vi "ProdaNG.Tree.TestSteps.Add.vi"(5 "Mode":T4, 6 "FileContent":T1, 7 "TestStepsTree":refnum<vi>, 8 "error in (no error)":errorcluster, 9 "units":T5[](array[typedef]), 10 "processStepId":i32, 11 "dbHandleIn":i32) -> (0 "error out":errorcluster, 1 "#changes":i32, 3 "dbHandle":i32)   [LabVIEW 2016]
doc: "This function returns a product structure for a product, which is identified by a part and a serial number.\nImportant information: The field 'individual' was taken over from the field 'allgemein' of the legacy data directly. Because of this most products have the value 0 further on and only a few the value 1. \nParameter:\nhandle is an Integer, which is returned by the function Login() at the creation of a new connection.\nwabcoPartId is the Id of the part.\nserialNumber is the serial number of the product for the part above.\nproduct is a pointer on a product structure, which is filled if the returncode is 0. The structure must be defined in the calling program.\n\nReturncodes:\n0 No error\n< 0 ORACLE Error code\n6 (ERROR_INVALID_HANDLE) in case of an invalid handle\n1403 Record does not exist"
uses:
  Controls/ProdaNG.UnitSimple.ctl
  ProdaNG.Tree.TestViewMode.ctl
  ProdaNG.File.Sequence.ctl
  ProdaNG.Tree.Fglb.Value.ctl
  ProdaNG.File.Step.ctl
  ProdaNG.Tree.Fglb.Data.ctl
  ProdaNG.Tree.Fglb.Element.ctl
  ProdaNG.Tree.Fglb.Action.ctl
  ProdaNG.Configurator.Glb.vi
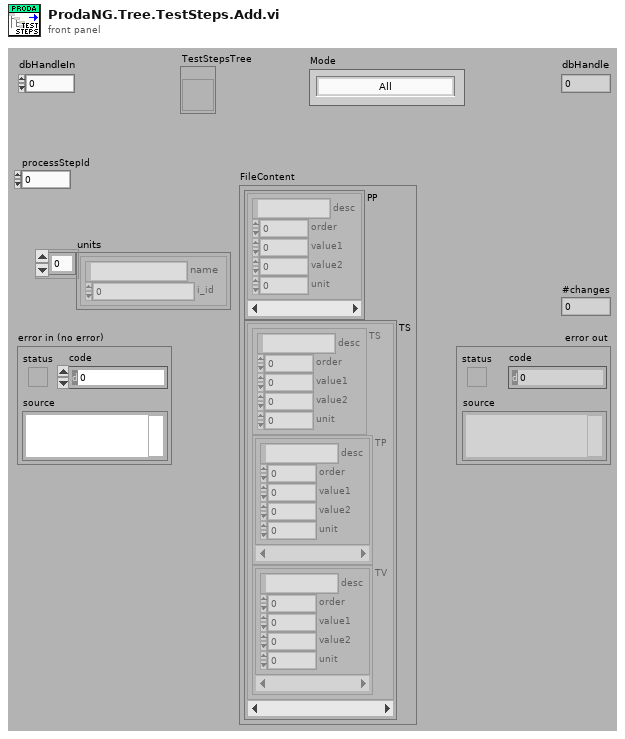
[diagram p1: front panel]
types:
  T1 = typedef "ProdaNG.File.Sequence.ctl" = cluster{"PP":T2[], "TS":T3[]}
  T2 = typedef "ProdaNG.Tree.Fglb.Value.ctl" = cluster{"desc":string, "order":i32, "value1":dbl, "value2":dbl, "unit":i32}
  T3 = typedef "ProdaNG.File.Step.ctl" = cluster{"TS":T2, "TP":T2[], "TV":T2[]}
  T4 = typedef "ProdaNG.Tree.TestViewMode.ctl" = enum16{"All", "Released", "Unreleased"}
  T5 = typedef "ProdaNG.UnitSimple.ctl" = cluster{"name":string, "i_id":i32}
  T6 = typedef "ProdaNG.Tree.Fglb.Action.ctl" = enum16{"init", "add", "get by row", "get by tag", "get by idx"}
  T7 = typedef "ProdaNG.Tree.Fglb.Element.ctl" = enum16{"-", "PP", "TS", "TP", "TV"}
  T8 = typedef "ProdaNG.Tree.Fglb.Data.ctl" = cluster{"tag":string, "row":i32, "element":T7, "idx1":i32, "idx2":i32, "file":bool}
  T9 = typedef "ProdaNG.TestStep.ctl" = cluster{"i_id":i32, "processStepId":i32, "testSequence":i32, "testOrder":i32, "mdReason":string, "mdUser":string, "mdTime":string, "description":string}
  T10 = typedef "ProdaNG.TestStepParam.ctl" = cluster{"i_id":i32, "testStepId":i32, "unitId":i32, "contentId":string, "previewId":string, "value":dbl, "valueText":string, "paramSequence":i32, "history":i32, "mdReason":string, "mdUser":string, "mdTime":string, "description":string}
  T11 = typedef "ProdaNG.TestValue.ctl" = cluster{"i_id":i32, "testStepId":i32, "releaseId":i32, "unitId":i32, "contentId":string, "previewId":string, "maximum":dbl, "minimum":dbl, "valueText":string, "testValueSequence":i32, "history":i32, "mdReason":string, "mdUser":string, "mdTime":string, "description":string}
  T12 = cluster{"TestStep":T9, "TestStepParams":T10[], "TestStepValues":T11[]}
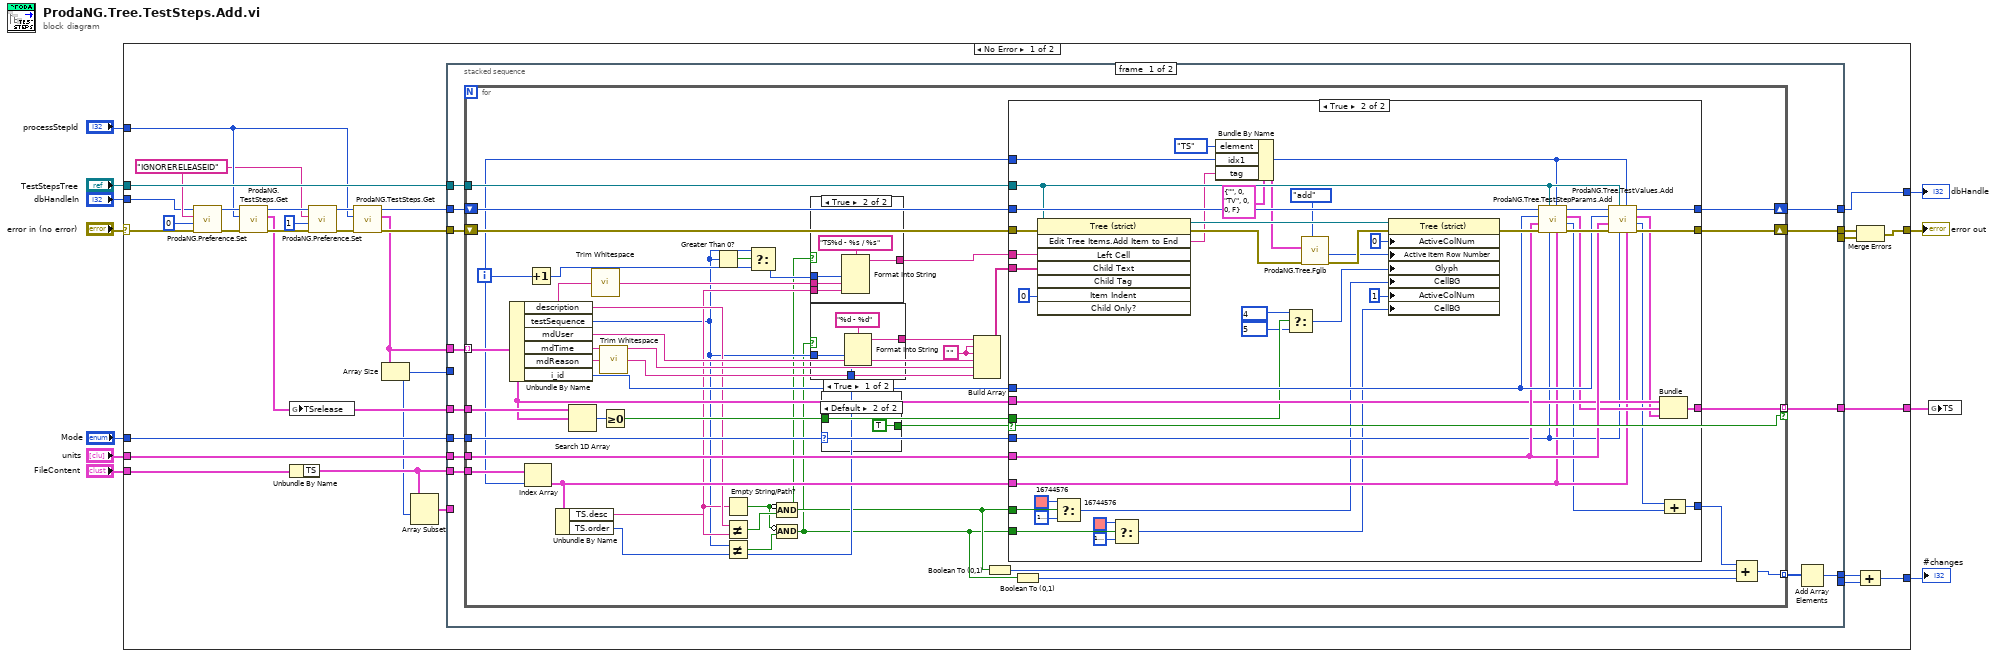
[diagram p0: block diagram]
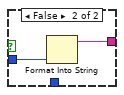
[diagram p2: hidden frame]
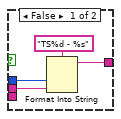
[diagram p3: hidden frame]
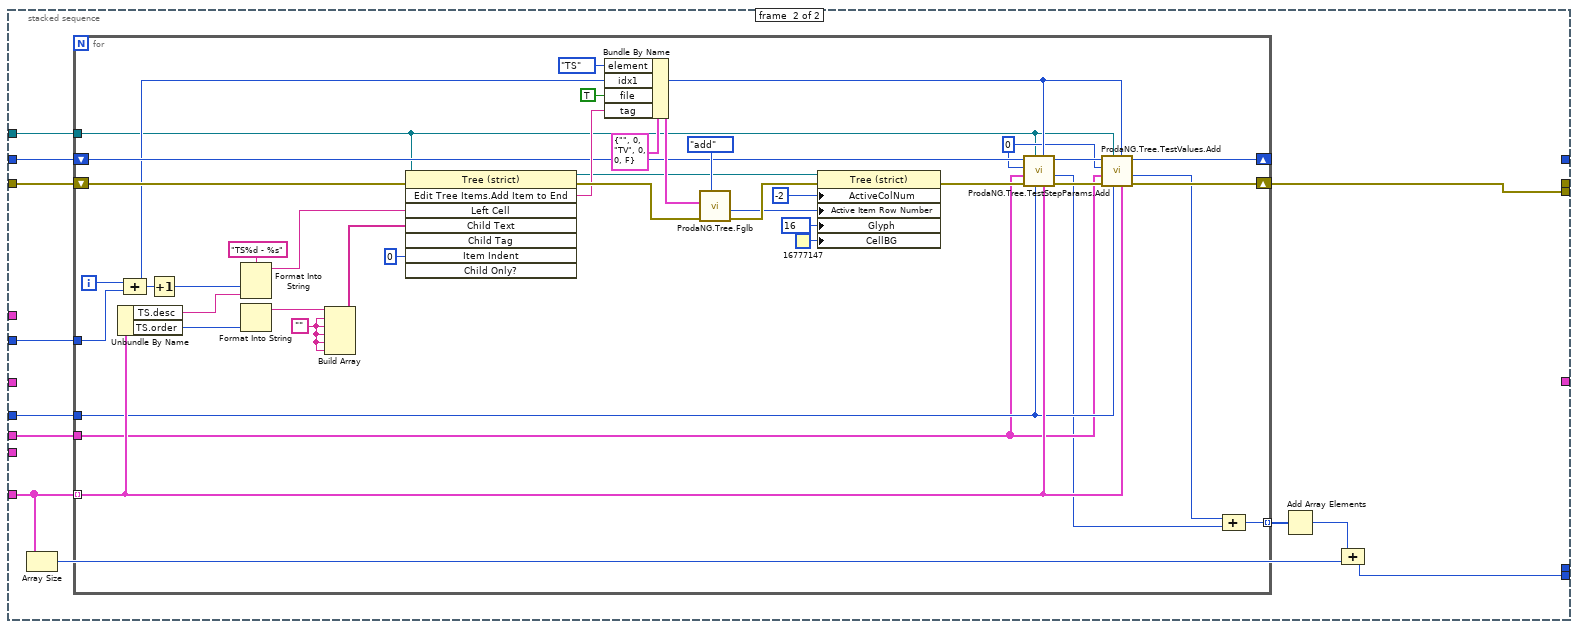
[diagram p6: hidden frame]
diagram:
  n1 = case shown="No Error" "error in (no error)" {
    selector: "error in (no error)" -> [w28 w215]
    tunnel: [w20 w215] -> w7
    tunnel: "dbHandleIn" -> [w25 w214]
    tunnel: [w36 w214] -> w9
    tunnel: "processStepId" -> [w27 _]
    tunnel: "TestStepsTree" -> [w40 _]
    tunnel: "units" -> [w38 _]
    tunnel: [w23 _] -> w4
    tunnel: "Mode" -> [w22 _]
    tunnel: "FileContent" -> [w21 _]
    tunnel: [w13 _] -> w1
    frame No Error {
      w26 = "IGNORERELEASEID" ("key")
      n2 = call "ProdaNG.Preference.Set.vi"("error in"=w28, "value"=0, "key"=w26, "dbHandleIn"=w25) -> ("dbHandle"=w32:i32)  [unwired: 6 in, 1 out]
      n3 = call "ProdaNG.TestSteps.Get.vi"("error in (no error)"=w28, "processStepId"=w27, "dbHandleIn"=w32) -> ("error out"=w31:errorcluster, "TestSteps"=w24:T9[], "dbHandle"=w33:i32)  [unwired: 6 in]
      n4 = global write "ProdaNG.Configurator.Glb.vi" "TSrelease"(w24) -> ()
      n5 = Unbundle By Name(w21) -> ("TS"=w18:T3[])
      n6 = call "ProdaNG.Preference.Set.vi"("error in"=w31, "value"=1, "key"=w26, "dbHandleIn"=w33) -> ("error out"=w30:errorcluster, "dbHandle"=w29:i32)  [unwired: 6 in]
      n7 = call "ProdaNG.TestSteps.Get.vi"("error in (no error)"=w30, "processStepId"=w27, "dbHandleIn"=w29) -> ("error out"=w41:errorcluster, "TestSteps"=w19:T9[], "dbHandle"=w39:i32)  [unwired: 6 in]
      n8 = Array Size(array=w19) -> (size(s)=w16:i32)
      n9 = Array Subset(array=w18, index=w16) -> (w17:T3[])  [unwired: 1 in]
      n10 = stacked-sequence {
        tunnel: w41 -> [w54 w173]
        tunnel: w40 -> [w53 w170]
        tunnel: w39 -> [w52 w171]
        tunnel: w38 -> [w51 w168]
        tunnel: w19 -> [w50 _]
        tunnel: [w49 _] -> w37
        tunnel: [w48 _] -> w36
        tunnel: w24 -> [w47 _]
        tunnel: [w46 _] -> w23
        tunnel: w22 -> [w45 w169]
        tunnel: w18 -> [w44 _]
        tunnel: w17 -> [_ w162]
        tunnel: w16 -> [_ w166]
        tunnel: [_ w172] -> w15
        tunnel: [w42 _] -> w14
        tunnel: [_ w164] -> w12
        frame #0 {
          n11 = for {
            shift-right: [w90] -> w49
            shift-left: w54 -> [w91]
            tunnel: w50 -> [w84] mode=indexing
            tunnel: w53 -> [w88]
            shift-right: [w77] -> w48
            shift-left: w52 -> [w89]
            tunnel: w51 -> [w85]
            tunnel: w47 -> [w87]
            tunnel: [w83] -> w46 mode=indexing if=w78
            tunnel: w45 -> [w76]
            tunnel: w44 -> [w73]
            tunnel: [w56] -> w43 mode=indexing
            i -> [w72]
            w81 = ""
            n12 = Unbundle By Name(w84) -> ("description"=w70:string, "testSequence"=w62:i32, "mdUser"=w94:string, "mdTime"=w95:string, "mdReason"=w92:string, "i_id"=w74:i32)
            n13 = Index Array(array=w73, index=w72) -> (element=w71:T3)
            n14 = Increment(x=w72) -> (x+1=w63:i32)
            n15 = Unbundle By Name(w71) -> ("TS.desc"=w66:string, "TS.order"=w65:i32)
            n16 = Search 1D Array(1D array=w87, element=w84) -> (index of element=w86:i32)  [unwired: 1 in]
            n17 = call <vilib>:"Trim Whitespace.vi"("string"=w70) -> ("trimmed string"=w82:string)  [unwired: 1 in]
            n18 = call <vilib>:"Trim Whitespace.vi"("string"=w92) -> ("trimmed string"=w75:string)  [unwired: 1 in]
            n19 = Greater Or Equal To 0?(x=w86) -> (x >= 0?=w79:bool)
            n20 = Greater Than 0?(x=w62) -> (x > 0?=w64:bool)
            n21 = Empty String/Path?(string/path=w66) -> (empty?=w68:bool)
            n22 = Not Equal?(x=w70, y=w66) -> (x != y?=w69:bool)
            n23 = Not Equal?(x=w62, y=w65) -> (x != y?=w67:bool)
            n24 = Select(t=w62, s=w64, f=w63) -> (s? t:f=w61:i32)
            n25 = Compound Arithmetic op=AND(invert w68, w69) -> (w58:bool)
            n26 = Compound Arithmetic op=AND(invert w68, w67) -> (w57:bool)
            n27 = case shown="True" w58 {
              tunnel: w61 -> [w105 w110]
              tunnel: w82 -> [w104 w109]
              tunnel: [w103 w108] -> w80
              tunnel: w66 -> [_ w107]
              frame False {
                n28 = Format Into String(format string="TS%d - %s", w105, w104) -> (resulting string=w103:string)  [unwired: 2 in, 1 out]
              }
              frame True {
                n29 = Format Into String(format string="TS%d - %s / %s", w110, w109, w107) -> (resulting string=w108:string)  [unwired: 2 in, 1 out]
              }
            }
            n30 = case shown="True" w57 {
              tunnel: [w100 w102] -> w96
              tunnel: w62 -> [w99 w101]
              tunnel: w65 -> [w97 _]
              frame True {
                n31 = Format Into String(format string="%d - %d", w99, w97) -> (resulting string=w100:string)  [unwired: 2 in, 1 out]
              }
              frame False {
                n32 = Format Into String(w101) -> (resulting string=w102:string)  [unwired: 3 in, 1 out]
              }
            }
            n33 = case shown="Default" w76 {
              tunnel: [w160 TRUE] -> w78
              tunnel: w79 -> [w160 _]
              frame "Released" {
              }
              frame Default {
              }
            }
            n34 = Build Array(w96, w81, w81, w94, w95, w75) -> (w93:string[])
            n35 = Boolean To (0,1)(Boolean=w58) -> (0, 1=w59:i16)
            n36 = case shown="True" w78 {
              tunnel: w93 -> [_ w159]
              tunnel: w91 -> [w113 w157]
              tunnel: [w113 w156] -> w90
              tunnel: w89 -> [w112 w153]
              tunnel: w88 -> [_ w151]
              tunnel: w74 -> [_ w150]
              tunnel: w85 -> [_ w149]
              tunnel: w84 -> [_ w148]
              tunnel: [_ w145] -> w83
              tunnel: w72 -> [_ w144]
              tunnel: w80 -> [_ w143]
              tunnel: w79 -> [_ w142]
              tunnel: [w112 w158] -> w77
              tunnel: w76 -> [_ w128]
              tunnel: w71 -> [_ w127]
              tunnel: w58 -> [_ w121]
              tunnel: w57 -> [_ w120]
              tunnel: [_ w114] -> w55
              frame False {
              }
              frame True {
                n37 = invoke on="Invoke Node" class="Tree (strict)" method="Edit Tree Items.Add Item to End"(reference=w151, error in=w157, "Left Cell"=w143, "Child Text"=w159, "Item Indent"=0 ("New Item Indentation")) -> (reference out=w140:refnum<vi>, error out=w133:errorcluster, "Edit Tree Items:Add Item to End"=w132:string)  [unwired: 3 in, 5 out]
                n38 = Select(t=u32 16744576, s=w121, f=u32 16777225) -> (s? t:f=w119:u32)
                n39 = Select(t=u32 16744576, s=w120, f=u32 16777225) -> (s? t:f=w117:u32)
                n40 = Bundle By Name(cluster=T8 {"tag"="", "row"=0, "element"=enum."TV", "idx1"=0, "idx2"=0, "file"=FALSE} ("entry in"), "element"=ProdaNG.Tree.Fglb.Element."TS", "idx1"=w144, "tag"=w132) -> (w135:T8)
                n41 = Select(t=4, s=w142, f=5) -> (s? t:f=w118:i32)
                n42 = call "ProdaNG.Tree.Fglb.vi"("Action (add)"=ProdaNG.Tree.Fglb.Action."add", "error in"=w133, "entry in"=w135) -> ("error out"=w139:errorcluster, "active row"=w137:i32)  [unwired: 6 in, 1 out]
                n43 = property class="Tree (strict)"(reference=w140, error in=w139, "ActiveColNum"=0 ("Active Cell:Active Column Number"), "Active Item Row Number"=w137, "Glyph"=w118, "CellBG"=w119, "ActiveColNum"=1 ("Active Cell:Active Column Number"), "CellBG"=w117) -> (error out=w152:errorcluster)  [unwired: 1 out]
                n44 = call "ProdaNG.Tree.TestStepParams.Add.vi"(4:"TS"=w127, 5:"TS"=w144, "Mode"=w128, "TestStepsTree"=w151, "error in (no error)"=w152, "units"=w149, "testStepId"=w150, "dbHandleIn"=w153) -> ("error out"=w154:errorcluster, "#changes"=w115:i32, "TestStepParams"=w147:T10[], "dbHandle"=w155:i32)
                n45 = call "ProdaNG.Tree.TestValues.Add.vi"(4:"TS"=w127, 5:"TS"=w144, "Mode"=w128, "TestStepsTree"=w151, "error in (no error)"=w154, "units"=w149, "testStepId"=w150, "dbHandleIn"=w155) -> ("error out"=w156:errorcluster, "#changes"=w116:i32, "TestStepValues"=w146:T11[], "dbHandle"=w158:i32)
                n46 = Bundle("TestStep"=w148, "TestStepParams"=w147, "TestStepValues"=w146) -> (w145:T12)  [unwired: 1 in]
                n47 = Compound Arithmetic op=ADD(w116, w115) -> (w114:i32)
              }
            }
            n48 = Boolean To (0,1)(Boolean=w57) -> (0, 1=w60:i16)
            n49 = Compound Arithmetic op=ADD(w55, w59, w60) -> (w56:i32)
          }
          n50 = Add Array Elements(numeric array=w43) -> (sum=w42:i32)
        }
        frame #1 {
          n51 = Array Size(array=w162) -> (size(s)=w163:i32)
          n52 = for {
            tunnel: w162 -> [w181] mode=indexing
            tunnel: w166 -> [w210]
            shift-right: [w185] -> w172
            shift-left: w173 -> [w200]
            shift-right: [w183] -> _
            shift-left: w171 -> [w184]
            tunnel: w170 -> [w177]
            tunnel: w169 -> [w180]
            tunnel: w168 -> [w179]
            tunnel: [w174] -> w167 mode=indexing
            i -> [w209]
            w178 = 0 ("testStepId")
            w196 = ""
            n53 = Unbundle By Name(w181) -> ("TS.desc"=w211:string, "TS.order"=w212:i32)
            n54 = Compound Arithmetic op=ADD(w209, w210) -> (w182:i32)
            n55 = Increment(x=w182) -> (x+1=w208:i32)
            n56 = Format Into String(format string="TS%d - %s", w208, w211) -> (resulting string=w198:string)  [unwired: 2 in, 1 out]
            n57 = Format Into String(w212) -> (resulting string=w197:string)  [unwired: 3 in, 1 out]
            n58 = Build Array(w197, w196, w196, w196, w196, w196) -> (w195:string[])
            n59 = invoke on="Invoke Node" class="Tree (strict)" method="Edit Tree Items.Add Item to End"(reference=w177, error in=w200, "Left Cell"=w198, "Child Text"=w195, "Item Indent"=0 ("New Item Indentation")) -> (reference out=w194:refnum<vi>, error out=w203:errorcluster, "Edit Tree Items:Add Item to End"=w202:string)  [unwired: 3 in, 5 out]
            n60 = Bundle By Name(cluster=T8 {"tag"="", "row"=0, "element"=enum."TV", "idx1"=0, "idx2"=0, "file"=FALSE} ("entry in"), "element"=ProdaNG.Tree.Fglb.Element."TS", "idx1"=w182, "file"=TRUE, "tag"=w202) -> (w205:T8)
            n61 = call "ProdaNG.Tree.Fglb.vi"("Action (add)"=ProdaNG.Tree.Fglb.Action."add", "error in"=w203, "entry in"=w205) -> ("error out"=w193:errorcluster, "active row"=w191:i32)  [unwired: 6 in, 1 out]
            n62 = property class="Tree (strict)"(reference=w194, error in=w193, "ActiveColNum"=-2 ("Active Cell:Active Column Number"), "Active Item Row Number"=w191, "Glyph"=16, "CellBG"=u32 16777147) -> (error out=w186:errorcluster)  [unwired: 1 out]
            n63 = call "ProdaNG.Tree.TestStepParams.Add.vi"(4:"TS"=w181, 5:"TS"=w182, "Mode"=w180, "TestStepsTree"=w177, "error in (no error)"=w186, "units"=w179, "testStepId"=w178, "dbHandleIn"=w184) -> ("error out"=w187:errorcluster, "#changes"=w175:i32, "dbHandle"=w188:i32)  [unwired: 1 out]
            n64 = call "ProdaNG.Tree.TestValues.Add.vi"(4:"TS"=w181, 5:"TS"=w182, "Mode"=w180, "TestStepsTree"=w177, "error in (no error)"=w187, "units"=w179, "testStepId"=w178, "dbHandleIn"=w188) -> ("error out"=w185:errorcluster, "#changes"=w176:i32, "dbHandle"=w183:i32)  [unwired: 1 out]
            n65 = Compound Arithmetic op=ADD(w176, w175) -> (w174:i32)
          }
          n66 = Add Array Elements(numeric array=w167) -> (sum=w165:i32)
          n67 = Compound Arithmetic op=ADD(w165, w163) -> (w164:i32)
        }
      }
      n68 = Merge Errors(w37, w15) -> (w20:errorcluster)
      n69 = Compound Arithmetic op=ADD(w14, w12) -> (w13:i32)
    }
    frame Error {
    }
  }
  "error out" <- w7
  "dbHandle" <- w9
  "#changes" <- w1
  n70 = global write "ProdaNG.Configurator.Glb.vi" "TS"(w4) -> ()
